vi "ZeroMQ_FOC.vi"() -> ()   [LabVIEW 2018]
uses:
  <vilib>/addons/zeromq/socket_type.ctl
  <vilib>/addons/zeromq/socket_options.ctl
  <vilib>/addons/zeromq/zeromq.lvlib
  <vilib>/addons/zeromq/zmq_socket.lvclass
  <vilib>/addons/zeromq/zmq_context.lvclass
panel:
  out "command":string
  in  "stop 3":bool
  out "error out 3":errorcluster
  out "error out 2":errorcluster
  out "message":string
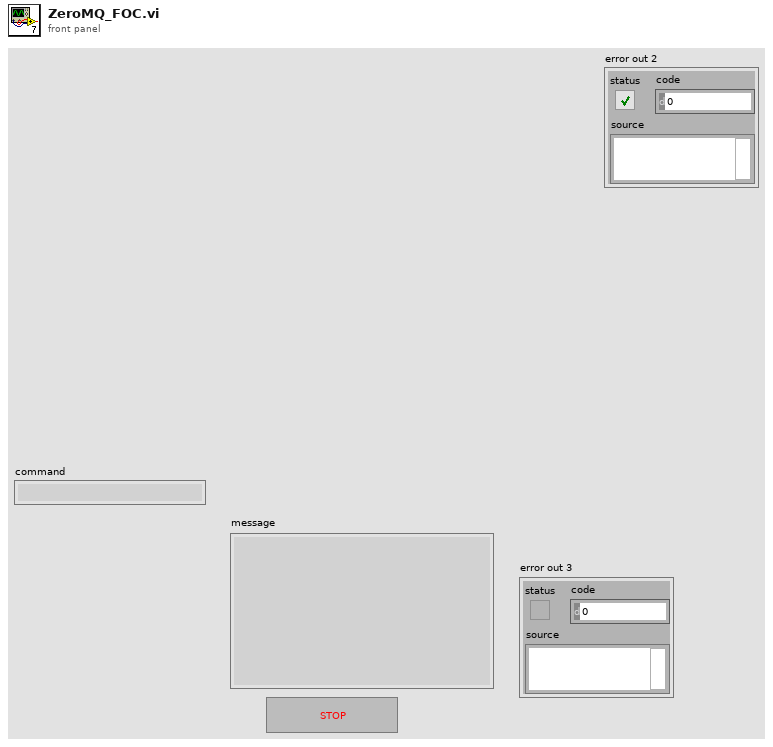
[diagram p1: front panel]
types:
  T1 = cluster{"ID":u32, "Address":string, "Service Name 1":string, "Service Name 2":string, "queue TX":refnum<queue>, "queue RX":refnum<queue>, "Port 1":u32, "Port 2":u32}
  T2 = typedef "zeromq.lvlib/socket_type.ctl" = enum8{"ZMQ_PAIR", "ZMQ_PUB", "ZMQ_SUB", "ZMQ_REQ", "ZMQ_REP", "ZMQ_DEALER", "ZMQ_ROUTER", "ZMQ_PULL", "ZMQ_PUSH", "ZMQ_XPUB", "ZMQ_XSUB", "ZMQ_STREAM", "ZMQ_SERVER", "ZMQ_CLIENT", "ZMQ_RADIO", "ZMQ_DISH", "ZMQ_GATHER", "ZMQ_SCATTER", "ZMQ_DGRAM"}
  T3 = typedef "zeromq.lvlib/socket_options.ctl" = enum8{"NONE", "ZMQ_HWM", "<2>", "ZMQ_SWAP", "ZMQ_AFFINITY", "ZMQ_ROUTING_ID", "ZMQ_SUBSCRIBE", "ZMQ_UNSUBSCRIBE", "ZMQ_RATE", "ZMQ_RECOVERY_IVL", "ZMQ_MCAST_LOOP", "ZMQ_SNDBUF", "ZMQ_RCVBUF", "ZMQ_RCVMORE", "ZMQ_FD", "ZMQ_EVENTS", "ZMQ_TYPE", "ZMQ_LINGER", "ZMQ_RECONNECT_IVL", "ZMQ_BACKLOG", "ZMQ_RECOVERY_IVL_MSEC", "ZMQ_RECONNECT_IVL_MAX", "ZMQ_MAXMSGSIZE", "ZMQ_SNDHWM", "ZMQ_RCVHWM", "ZMQ_MULTICAST_HOPS", "<26>", "ZMQ_RCVTIMEO", "ZMQ_SNDTIMEO", "<29>", "<30>", "ZMQ_IPV4ONLY", "ZMQ_LAST_ENDPOINT", "ZMQ_ROUTER_MANDATORY", "ZMQ_TCP_KEEPALIVE", "ZMQ_TCP_KEEPALIVE_CNT", "ZMQ_TCP_KEEPALIVE_IDLE", "ZMQ_TCP_KEEPALIVE_INTVL", "ZMQ_TCP_ACCEPT_FILTER", "ZMQ_IMMEDIATE", "ZMQ_XPUB_VERBOSE", "ZMQ_ROUTER_RAW", "ZMQ_IPV6", "ZMQ_MECHANISM", "ZMQ_PLAIN_SERVER", "ZMQ_PLAIN_USERNAME", "ZMQ_PLAIN_PASSWORD", "ZMQ_CURVE_SERVER", "ZMQ_CURVE_PUBLICKEY", "ZMQ_CURVE_SECRETKEY", "ZMQ_CURVE_SERVERKEY", "ZMQ_PROBE_ROUTER", "ZMQ_REQ_CORRELATE", "ZMQ_REQ_RELAXED", "ZMQ_CONFLATE", "ZMQ_ZAP_DOMAIN", "ZMQ_ROUTER_HANDOVER", "ZMQ_TOS", "ZMQ_IPC_FILTER_PID", "ZMQ_IPC_FILTER_UID", "ZMQ_IPC_FILTER_GID", "ZMQ_CONNECT_ROUTING_ID", "ZMQ_GSSAPI_SERVER", "ZMQ_GSSAPI_PRINCIPAL", "ZMQ_GSSAPI_SERVICE_PRINCIPAL", "ZMQ_GSSAPI_PLAINTEXT", "ZMQ_HANDSHAKE_IVL", "<67>", "ZMQ_SOCKS_PROXY", "ZMQ_XPUB_NODROP", "ZMQ_BLOCKY", "ZMQ_XPUB_MANUAL", "ZMQ_XPUB_WELCOME_MSG", "ZMQ_STREAM_NOTIFY", "ZMQ_INVERT_MATCHING", "ZMQ_HEARTBEAT_IVL", "ZMQ_HEARTBEAT_TTL", "ZMQ_HEARTBEAT_TIMEOUT", "ZMQ_XPUB_VERBOSER", "ZMQ_CONNECT_TIMEOUT", "ZMQ_TCP_MAXRT", "ZMQ_THREAD_SAFE", "<82>", "<83>", "ZMQ_MULTICAST_MAXTPDU", "ZMQ_VMCI_BUFFER_SIZE", "ZMQ_VMCI_BUFFER_MIN_SIZE", "ZMQ_VMCI_BUFFER_MAX_SIZE", "ZMQ_VMCI_CONNECT_TIMEOUT", "ZMQ_USE_FD", "ZMQ_GSSAPI_PRINCIPAL_NAMETYPE", "ZMQ_GSSAPI_SERVICE_PRINCIPAL_NAMETYPE", "ZMQ_BINDTODEVICE", "ZMQ_ZAP_ENFORCE_DOMAIN", "ZMQ_LOOPBACK_FASTPATH", "ZMQ_METADATA", "ZMQ_MULTICAST_LOOP", "ZMQ_ROUTER_NOTIFY"}
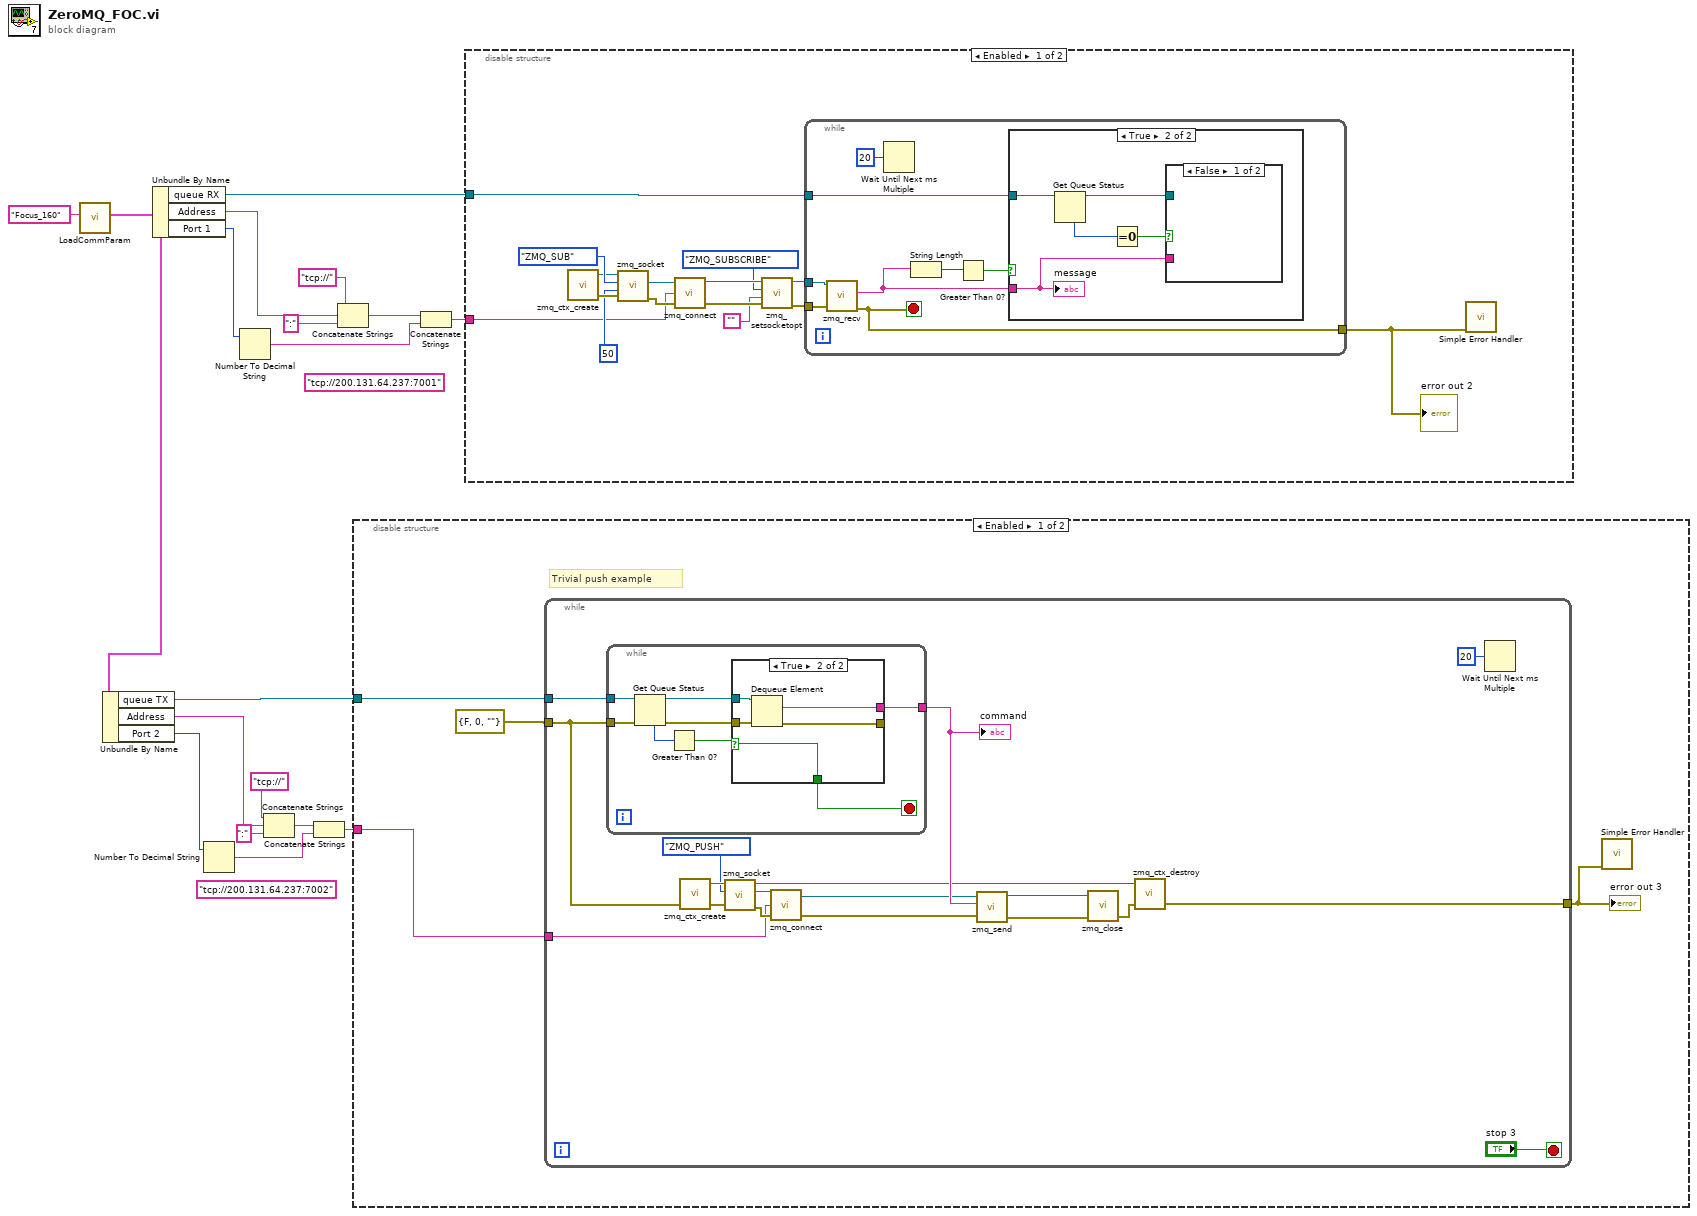
[diagram p0: block diagram]
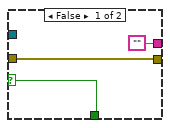
[diagram p2: hidden frame]
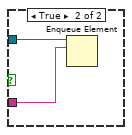
[diagram p5: hidden frame]
diagram:
  (unwired) "tcp://200.131.64.237:7002" ("endpoint")
  (unwired) "tcp://200.131.64.237:7001" ("endpoint")
  n1 = call "LoadCommParam.vi"("section name"="Focus_160") -> ("output cluster"=w1:T1)  [unwired: 10 in]
  n2 = Unbundle By Name(w1) -> ("queue TX"=w10:refnum<queue>, "Address"=w5:string, "Port 2"=w4:u32)
  n3 = Unbundle By Name(w1) -> ("queue RX"=w2:refnum<queue>, "Address"=w17:string, "Port 1"=w16:u32)
  n4 = Number To Decimal String(number=w4) -> (decimal integer string=w9:string)  [unwired: 1 in]
  n5 = Number To Decimal String(number=w16) -> (decimal integer string=w15:string)  [unwired: 1 in]
  n6 = Concatenate Strings("tcp://" ("string"), w5, ":" ("string")) -> (w8:string)
  n7 = Concatenate Strings(w8, w9) -> (w3:string)
  n8 = Concatenate Strings("tcp://" ("string"), w17, ":" ("string")) -> (w14:string)
  n9 = disable-structure shown="Enabled" {
    disable-tunnel: w10 -> [w21 _]
    disable-tunnel: w3 -> [w20 _]
    frame Enabled {
      # "Trivial push example"
      n10 = while {
        tunnel: w21 -> [w40]
        tunnel: errorcluster {"status"=FALSE, "code"=0, "source"=""} ("error out") -> [w24]
        tunnel: [w29] -> w22
        tunnel: w20 -> [w25]
        stop <- "stop 3" stop-if-true
        n11 = while {
          tunnel: w40 -> [w47]
          tunnel: w24 -> [w46]
          tunnel: [w42] -> w39
          stop <- w41 stop-if-true
          n12 = Get Queue Status(queue=w47, error in (no error)=w46) -> (queue out=w43:refnum<queue>, error out=w44:errorcluster, # elements in queue=w48:i32)  [unwired: 1 in, 5 out]
          n13 = Greater Than 0?(x=w48) -> (x > 0?=w45:bool)
          n14 = case shown="True" w45 {
            selector: w45 -> [w49 w52]
            tunnel: w44 -> [w51 w56]
            tunnel: w43 -> [_ w55]
            tunnel: [w51 w54] -> _
            tunnel: ["" w53] -> w42
            tunnel: [w49 w52] -> w41
            frame False {
            }
            frame True {
              n15 = Dequeue Element(queue=w55, error in (no error)=w56) -> (element=w53:string, error out=w54:errorcluster)  [unwired: 1 in, 2 out]
            }
          }
        }
        "command" <- w39
        n16 = call <vilib>:"zmq_ctx_create.vi"("error in"=w24) -> ("error out"=w34:errorcluster, "context out"=w37:refnum<class "zmq_context.lvclass">)  [unwired: 3 in]
        n17 = call <vilib>:"zmq_socket.vi"("error in"=w34, "socket type"=socket_type."ZMQ_PUSH", "context in"=w37) -> ("error out"=w36:errorcluster, "socket out"=w35:refnum<class "zmq_socket.lvclass">, "context out"=w28:refnum<class "zmq_context.lvclass">)  [unwired: 2 in]
        n18 = call <vilib>:"zmq_connect.vi"("error in"=w36, "endpoint"=w25, "socket in"=w35) -> ("error out"=w31:errorcluster, "socket out"=w32:refnum<class "zmq_socket.lvclass">)  [unwired: 1 in]
        n19 = call <vilib>:"zmq_send.vi"("error in"=w31, "data"=w39, "socket in"=w32) -> ("error out"=w26:errorcluster, "socket out"=w27:refnum<class "zmq_socket.lvclass">)  [unwired: 4 in]
        n20 = call <vilib>:"zmq_close.vi"("error in"=w26, "socket"=w27) -> ("error out"=w30:errorcluster)  [unwired: 3 in]
        n21 = call <vilib>:"zmq_ctx_destroy.vi"("error in"=w30, "context in"=w28) -> ("error out"=w29:errorcluster)  [unwired: 3 in]
        n22 = Wait Until Next ms Multiple(millisecond multiple=u32 20) -> ()  [unwired: 1 out]
      }
      "error out 3" <- w22
      n23 = call <vilib>:"Simple Error Handler.vi"("error in (no error)"=w22) -> ()  [unwired: 4 in, 5 out]
    }
    frame Disabled {
    }
  }
  n24 = Concatenate Strings(w14, w15) -> (w11:string)
  n25 = disable-structure shown="Enabled" {
    disable-tunnel: w2 -> [w58 _]
    disable-tunnel: w11 -> [w57 _]
    frame Enabled {
      n26 = call <vilib>:"zmq_ctx_create.vi"() -> ("error out"=w70:errorcluster, "context out"=w60:refnum<class "zmq_context.lvclass">)  [unwired: 4 in]
      n27 = call <vilib>:"zmq_socket.vi"("error in"=w70, "linger (ms)"=50, "socket type"=socket_type."ZMQ_SUB", "context in"=w60) -> ("error out"=w69:errorcluster, "socket out"=w61:refnum<class "zmq_socket.lvclass">)  [unwired: 1 in, 1 out]
      n28 = call <vilib>:"zmq_connect.vi"("error in"=w69, "endpoint"=w57, "socket in"=w61) -> ("error out"=w67:errorcluster, "socket out"=w68:refnum<class "zmq_socket.lvclass">)  [unwired: 1 in]
      n29 = call <vilib>:"zmq_setsocketopt.vi"("error in"=w67, "value"="", "option"=socket_options."ZMQ_SUBSCRIBE", "socket in"=w68) -> ("error out"=w66:errorcluster, "socket out"=w65:refnum<class "zmq_socket.lvclass">)  [unwired: 2 in]
      n30 = while {
        tunnel: w65 -> [w77]
        tunnel: w66 -> [w79]
        tunnel: [w78] -> w62
        tunnel: w58 -> [w74]
        stop <- w78 stop-if-true
        n31 = call <vilib>:"zmq_recv.vi"("error in"=w79, "socket in"=w77) -> ("error out"=w78:errorcluster, "data"=w73:string)  [unwired: 3 in, 3 out]
        n32 = Wait Until Next ms Multiple(millisecond multiple=u32 20) -> ()  [unwired: 1 out]
        n33 = String Length(string=w73) -> (length=w76:i32)
        n34 = Greater Than 0?(x=w76) -> (x > 0?=w75:bool)
        n35 = case shown="True" w75 {
          tunnel: w74 -> [_ w83]
          tunnel: w73 -> [_ w80]
          frame False {
          }
          frame True {
            n36 = Get Queue Status(queue=w83) -> (queue out=w81:refnum<queue>, # elements in queue=w84:i32)  [unwired: 2 in, 6 out]
            n37 = Equal To 0?(x=w84) -> (x = 0?=w82:bool)
            n38 = case shown="False" w82 {
              tunnel: w81 -> [_ w86]
              tunnel: w80 -> [_ w85]
              frame False {
              }
              frame True {
                n39 = Enqueue Element(queue=w86, element=w85) -> ()  [unwired: 2 in, 3 out]
              }
            }
            "message" <- w80
          }
        }
      }
      "error out 2" <- w62
      n40 = call <vilib>:"Simple Error Handler.vi"("error in (no error)"=w62) -> ()  [unwired: 4 in, 5 out]
    }
    frame Disabled {
    }
  }
